vi "WSVCAP SHL Host TL RFFE Read - Single DUT.vi"(0 "Data Out":string, 11 "error in":errorcluster, 12 "Log (T)":bool=TRUE, 13 "DUT":T2, 14 "FPGA":T1) -> (4 "Data In":string, 15 "error out":errorcluster)   [LabVIEW 2012]
uses:
  Type Defs/WSVCAP SHL DUT Number Enum.ctl
  Type Defs/WSVCAP SHL I2C FPGA Enum.ctl
panel:
  out "RFFE Data In":u8[][](array[numeric]) format="%02x"
  out "Socket Mask":u64=1 format="%02x"
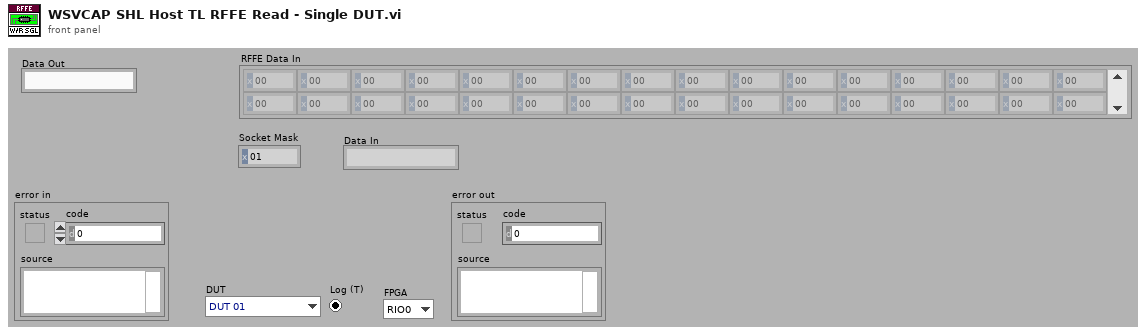
[diagram p1: front panel]
types:
  T1 = typedef "WSVCAP SHL I2C FPGA Enum.ctl" = enum16{"RIO0", "RIO1"}
  T2 = typedef "WSVCAP SHL DUT Number Enum.ctl" = enum16{"DUT 01", "DUT 02", "DUT 03", "DUT 04", "DUT 05", "DUT 06", "DUT 07", "DUT 08", "DUT 09", "DUT 10", "DUT 11", "DUT 12", "DUT 13", "DUT 14", "DUT 15", "DUT 16", "DUT 17", "DUT 18", "DUT 19", "DUT 20", "DUT 21", "DUT 22", "DUT 23", "DUT 24", "DUT 25", "DUT 26", "DUT 27", "DUT 28", "DUT 29", "DUT 30", "DUT 31", "DUT 32", "DUT 33", "DUT 34", "DUT 35", "DUT 36"}
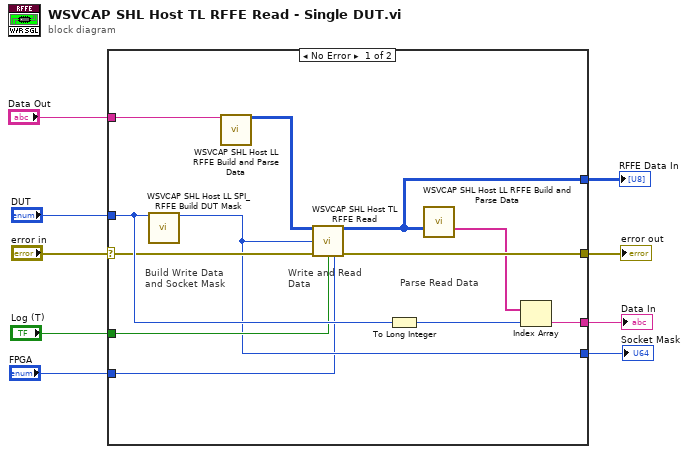
[diagram p0: block diagram]
diagram:
  n1 = case shown="No Error" "error in" {
    selector: "error in" -> [w20 _]
    tunnel: [w19 _] -> w9
    tunnel: "DUT" -> [w21 _]
    tunnel: [w17 _] -> w6
    tunnel: [w13 _] -> w5
    tunnel: [w14 _] -> w4
    tunnel: "Log (T)" -> [w16 _]
    tunnel: "Data Out" -> [w12 _]
    tunnel: "FPGA" -> [w10 _]
    frame No Error {
      # "Parse Read Data"
      # "Write and Read\nData"
      # "Build Write Data and Socket Mask"
      n2 = call "WSVCAP SHL Host LL SPI_RFFE Build DUT Mask.vi"("DUT"=w21) -> ("Socket Mask [U64]"=w13:u64)  [unwired: 13 in, 1 out]
      n3 = call "WSVCAP SHL Host LL RFFE Build and Parse Data.vi"("Data Out"=w12) -> ("RFFE Data Out [U8]"=w11:u8[][])  [unwired: 11 in, 3 out]
      n4 = call "WSVCAP SHL Host TL RFFE Read.vi"("Write Data In [DUT Ordered]"=w11, "Socket Mask"=w13, "error in"=w20, "Log (T)"=w16, "FPGA"=w10) -> ("Read Data Out"=w14:u8[][], "error out"=w19:errorcluster)  [unwired: 9 in]
      n5 = To Long Integer(number=w21) -> (32bit integer=w18:i32)
      n6 = call "WSVCAP SHL Host LL RFFE Build and Parse Data.vi"("RFFE Data In [U8]"=w14) -> ("RFFE Data In"=w15:string[])  [unwired: 11 in, 3 out]
      n7 = Index Array(array=w15, index=w18) -> (element=w17:string)
    }
    frame Error {
    }
  }
  "error out" <- w9
  "Socket Mask" <- w5
  "Data In" <- w6
  "RFFE Data In" <- w4
